vi "Log Event.vi"(8 "error in (no error)":errorcluster caption="错误输入（无错误）", 10 "Event Text":string, 11 "ControlPanel输入":refnum<class "ControlPanel.lvclass">) -> (0 "error out":errorcluster caption="错误输出", 3 "ControlPanel输出":refnum<class "ControlPanel.lvclass">)   [LabVIEW 2014, in "ControlPanel.lvlib" / "ControlPanel.lvclass"]
uses:
  ControlPanel.lvclass
  ControlPanel.lvclass/ControlPanel.ctl
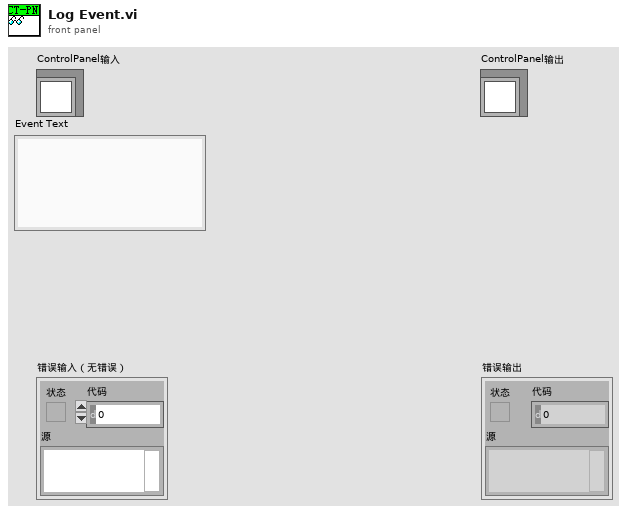
[diagram p1: front panel]
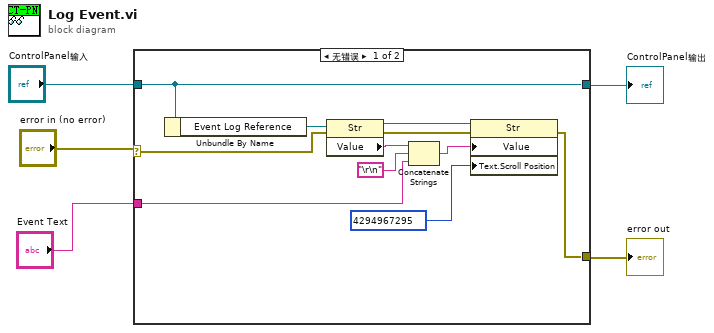
[diagram p0: block diagram]
diagram:
  n1 = case shown="无错误" "error in (no error)" {
    selector: "error in (no error)" -> [w7 w17]
    tunnel: [w6 w17] -> w5
    tunnel: [w16 w18] -> w3
    tunnel: "ControlPanel输入" -> [w16 w18]
    tunnel: "Event Text" -> [w8 _]
    frame No Error {
      n2 = Unbundle By Name(w16) -> ("Event Log Reference"=w9:refnum<vi>)
      n3 = property class="Str"(reference=w9, error in=w7) -> (reference out=w13:refnum<vi>, error out=w12:errorcluster, "Value"=w15:string)
      n4 = Concatenate Strings(w15, "\r\n", w8) -> (w11:string)
      n5 = property class="Str"(reference=w13, error in=w12, "Value"=w11, "Text.Scroll Position"=u32 4294967295) -> (error out=w6:errorcluster)  [unwired: 1 out]
    }
    frame Error {
    }
  }
  "error out" <- w5
  "ControlPanel输出" <- w3
